vi "wsHandlerEngine.vi"(8 "error in (no error)":errorcluster, 11 "References":T1) -> (0 "error out":errorcluster)   [LabVIEW 2018, in "HASS-LV-WS_integration.lvlib"]
uses:
  HASS-LV-WS_integration.lvlib
  TypeDef/ReferencesTypeDef.ctl
  TypeDef/QueueTypeDef.ctl
  TypeDef/EventTypeDef.ctl
  TypeDef/registeredEventTypeDef.ctl
  <vilib>/MediaMongrels Ltd/WebSockets/WebSockets/WebSockets.lvlib
panel:
  out "error live":errorcluster
  out "eventMsgIDs":string[](array[string])
  out "Log":string
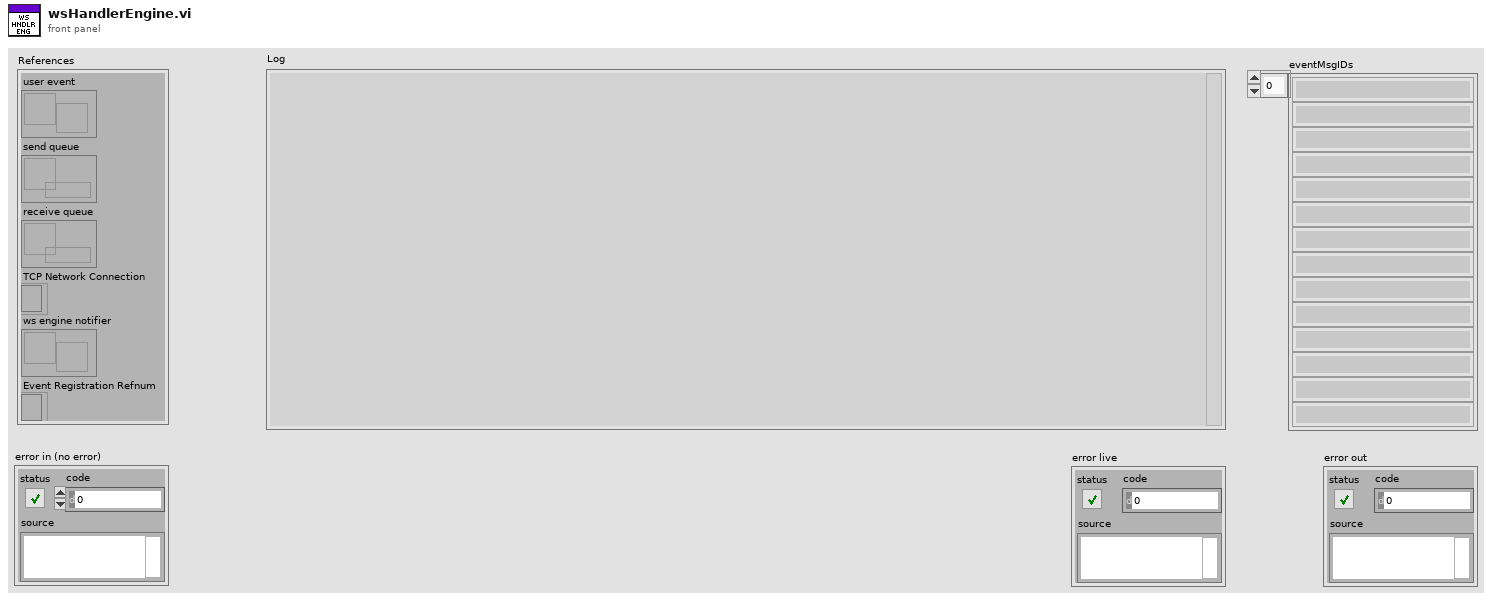
[diagram p1: front panel]
types:
  T1 = typedef "HASS-LV-WS_integration.lvlib/ReferencesTypeDef.ctl" = cluster{"user event":refnum<user-event>, "send queue":refnum<queue>, "receive queue":refnum<queue>, "TCP Network Connection":refnum<k5>, "ws engine notifier ":refnum<notifier>, "Event Registration Refnum":refnum<event-registration>}
  T2 = typedef "HASS-LV-WS_integration.lvlib/EventTypeDef.ctl" = cluster{"Data":variant, "Command":string}
  T3 = typedef "HASS-LV-WS_integration.lvlib/registeredEventTypeDef.ctl" = enum16{"Init", "Register", "Unregister", "Get MSG ID", "Get Event Name", "Get All Events"}
  T4 = typedef "HASS-LV-WS_integration.lvlib/QueueTypeDef.ctl" = cluster{"Data":variant, "Command":string}
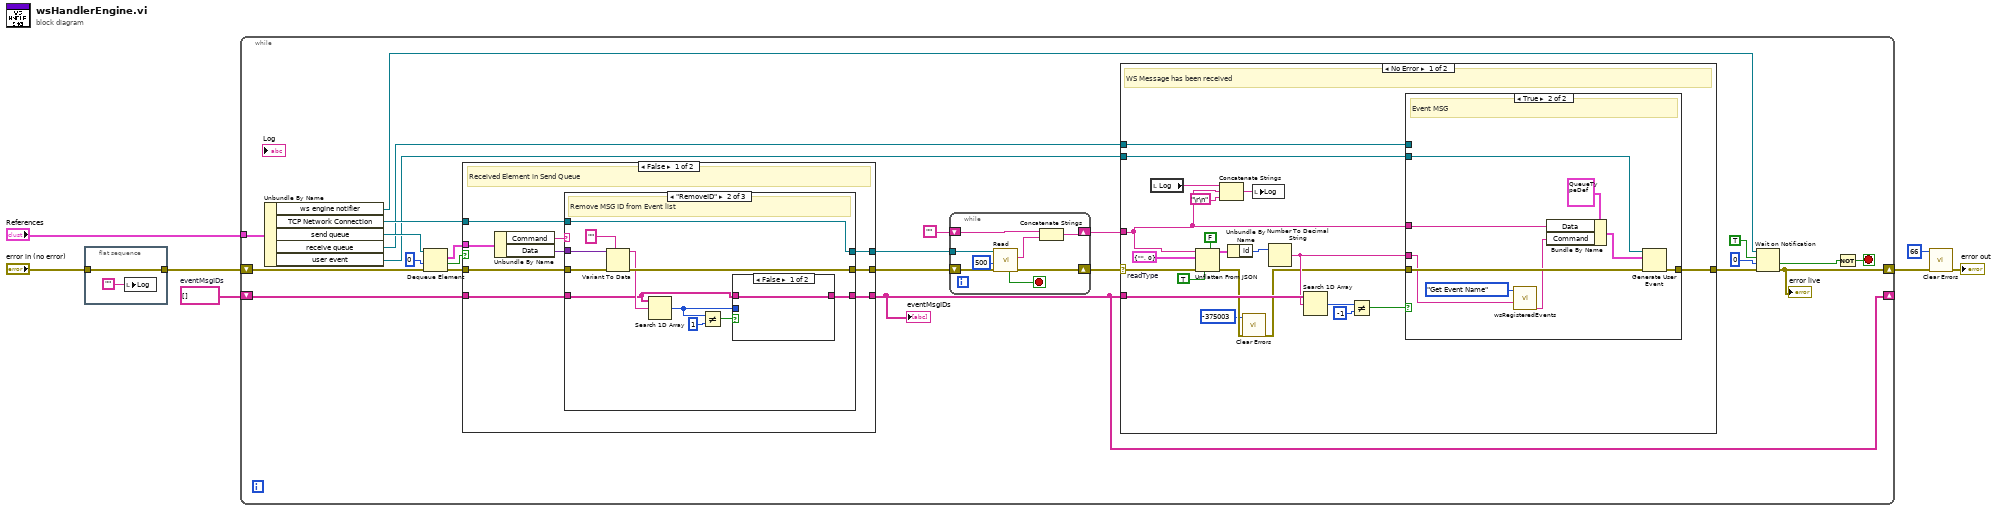
[diagram p0: block diagram]
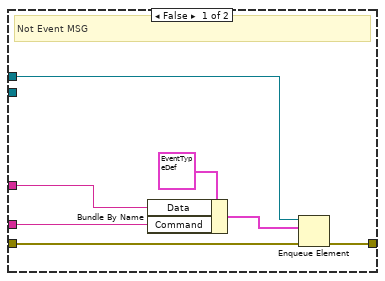
[diagram p2: hidden frame]
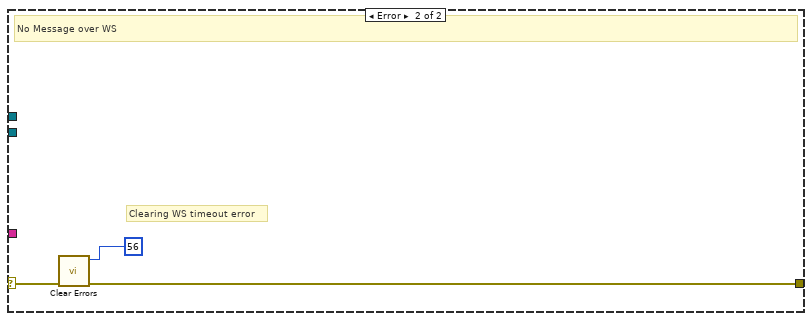
[diagram p3: hidden frame]
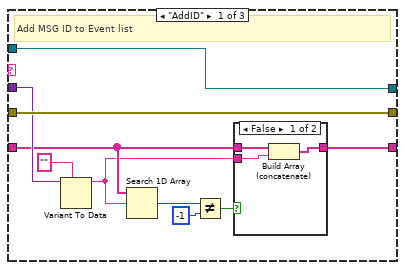
[diagram p4: hidden frame]
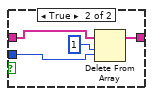
[diagram p6: hidden frame]
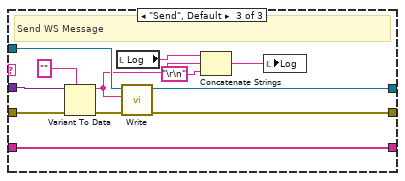
[diagram p7: hidden frame]
diagram:
  w7 = string[] []  # eventMsgIDs
  n1 = flat-sequence {
    tunnel: "error in (no error)" -> [w9]
    tunnel: [w9] -> w4
    frame #0 {
      n2 = local write "Log"("") -> ()
    }
  }
  n3 = while {
    tunnel: "References" -> [w33]
    shift-right: [w21] -> _
    shift-left: w7 -> [w23]
    shift-right: [w13] -> w3
    shift-left: w4 -> [w30]
    stop <- w15 stop-if-true
    n4 = Unbundle By Name(w33) -> ("ws engine notifier"=w18:refnum<notifier>, "TCP Network Connection"=w29:refnum<k5>, "send queue"=w32:refnum<queue>, "receive queue"=w19:refnum<queue>, "user event"=w20:refnum<user-event>)
    n5 = Dequeue Element(queue=w32, timeout in ms (-1)=0, error in (no error)=w30) -> (element=w26:T2, timed out?=w27:bool, error out=w28:errorcluster)  [unwired: 1 out]
    n6 = case shown="False" w27 {
      tunnel: w29 -> [w90 w134]
      tunnel: w28 -> [w89 w135]
      tunnel: w26 -> [w88 _]
      tunnel: [w86 w135] -> w25
      tunnel: [w85 w134] -> w24
      tunnel: w23 -> [w83 w133]
      tunnel: [w82 w133] -> w21
      frame False {
        # "Received Element in Send Queue"
        n7 = Unbundle By Name(w88) -> ("Command"=w84:string, "Data"=w87:variant)
        n8 = case shown="\"RemoveID\"" w84 {
          tunnel: w90 -> [w100 w115 w132]
          tunnel: w89 -> [w99 w113 w125]
          tunnel: w87 -> [w98 w114 w131]
          tunnel: [w99 w112 w129] -> w86
          tunnel: [w100 w115 w128] -> w85
          tunnel: w83 -> [w94 w109 w127]
          tunnel: [w91 w108 w127] -> w82
          frame "AddID" {
            # "Add MSG ID to Event list"
            n9 = Variant To Data(type="", Variant=w98) -> (data=w93:string)  [unwired: 1 in, 1 out]
            n10 = Search 1D Array(1D array=w94, element=w93) -> (index of element=w96:i32)  [unwired: 1 in]
            n11 = Not Equal?(x=w96, y=-1) -> (x != y?=w92:bool)
            n12 = case shown="False" w92 {
              tunnel: w94 -> [w103 w104]
              tunnel: w93 -> [w102 _]
              tunnel: [w101 w104] -> w91
              frame False {
                n13 = Build Array (concatenate)(w103, w102) -> (w101:string[])
              }
              frame True {
              }
            }
          }
          frame "RemoveID" {
            # "Remove MSG ID from Event list"
            n14 = Variant To Data(error in=w113, type="", Variant=w114) -> (data=w111:string, error out=w112:errorcluster)
            n15 = Search 1D Array(1D array=w109, element=w111) -> (index of element=w107:i32)  [unwired: 1 in]
            n16 = Not Equal?(x=w107, y=1) -> (x != y?=w105:bool)
            n17 = case shown="False" w105 {
              tunnel: w109 -> [w116 w120]
              tunnel: [w116 w119] -> w108
              tunnel: w107 -> [_ w117]
              frame False {
              }
              frame True {
                n18 = Delete From Array(array=w120, length=1, index=w117) -> (array with subset deleted=w119:string[])  [unwired: 1 out]
              }
            }
          }
          frame "Send", Default {
            # "Send WS Message"
            n19 = Variant To Data(error in=w125, type="", Variant=w131) -> (data=w121:string, error out=w126:errorcluster)
            n20 = local read "Log"() -> (w123:string)
            n21 = call <vilib>:"Write.vi"("error in (no error)"=w126, "Data"=w121, "WebSocket Connection in"=w132) -> ("error out"=w129:errorcluster, "WebSocket Connection out"=w128:refnum<k5>)  [unwired: 7 in]
            n22 = Concatenate Strings(w123, w121, "\r\n") -> (w124:string)
            n23 = local write "Log"(w124) -> ()
          }
        }
      }
      frame True {
        # "Send Queue Timed Out"
      }
    }
    "eventMsgIDs" <- w21
    n24 = while {
      tunnel: w24 -> [w40]
      shift-right: [w38] -> w22
      shift-left: w25 -> [w41]
      shift-right: [w36] -> w10
      shift-left: "" -> [w35]
      stop <- w37 stop-if-true
      n25 = call <vilib>:"Read.vi"("error in (no error)"=w41, "timeout ms (5000)"=500, "WebSocket Connection in"=w40) -> ("error out"=w38:errorcluster, "Data"=w34:string, "Finished?"=w37:bool)  [unwired: 4 in, 2 out]
      n26 = Concatenate Strings(w35, w34) -> (w36:string)
    }
    n27 = case shown="No Error" w22 {
      selector: w22 -> [w60 w81]
      tunnel: w10 -> [w49 _]
      tunnel: [w53 w80] -> w14
      tunnel: w21 -> [w59 _]
      tunnel: w20 -> [w55 _]
      tunnel: w19 -> [w54 _]
      frame No Error {
        w62 = cluster{"type":string, "id":i32} {"type"="", "id"=0}  # readType
        # "WS Message has been received"
        n28 = local read "Log"() -> (w51:string)
        n29 = Unflatten From JSON(enable LabVIEW extensions? (T)=FALSE, JSON string=w49, type and defaults=w62, default null elements? (F)=TRUE, error in (no error)=w60) -> (value=w61:cluster{"type":string, "id":i32}, error out=w44:errorcluster)  [unwired: 2 in]
        n30 = Concatenate Strings(w51, w49, "\r\n") -> (w50:string)
        n31 = Unbundle By Name(w61) -> ("id"=w48:i32)
        n32 = call <vilib>:"Clear Errors.vi"("error in (no error)"=w44, "specific error code to clear (0: all)"=-375003) -> ("error out"=w43:errorcluster)  [unwired: 4 in, 1 out]
        n33 = local write "Log"(w50) -> ()
        n34 = Number To Decimal String(number=w48) -> (decimal integer string=w47:string)  [unwired: 1 in]
        n35 = Search 1D Array(1D array=w59, element=w47) -> (index of element=w58:i32)  [unwired: 1 in]
        n36 = Not Equal?(x=w58, y=-1) -> (x != y?=w56:bool)
        n37 = case shown="True" w56 {
          tunnel: w55 -> [_ w78]
          tunnel: w43 -> [w68 w77]
          tunnel: w47 -> [w63 w72]
          tunnel: w54 -> [w69 _]
          tunnel: [w67 w74] -> w53
          tunnel: w49 -> [w64 w73]
          frame False {
            # "Not Event MSG"
            n38 = Bundle By Name(cluster=T2 {"Data"=variant, "Command"=""} ("element"), "Data"=w64, "Command"=w63) -> (w65:T2)
            n39 = Enqueue Element(queue=w69, element=w65, error in (no error)=w68) -> (error out=w67:errorcluster)  [unwired: 1 in, 2 out]
          }
          frame True {
            # "Event MSG"
            n40 = call "wsRegisteredEvents.vi"("msgID"=w72, "Action"=registeredEventTypeDef."Get Event Name") -> ("Event Name"=w71:string)  [unwired: 6 in, 3 out]
            n41 = Bundle By Name(cluster=T4 {"Data"=variant, "Command"=""} ("event data"), "Data"=w73, "Command"=w71) -> (w75:T4)
            n42 = Generate User Event(user event=w78, event data cluster=w75, error in=w77) -> (error out=w74:errorcluster)  [unwired: 1 in, 1 out]
          }
        }
      }
      frame Error {
        # "Clearing WS timeout error"
        # "No Message over WS"
        n43 = call <vilib>:"Clear Errors.vi"("error in (no error)"=w81, "specific error code to clear (0: all)"=56) -> ("error out"=w80:errorcluster)  [unwired: 4 in, 1 out]
      }
    }
    n44 = Wait on Notification(notifier=w18, ignore previous (F)=TRUE, timeout in ms (-1)=0, error in (no error)=w14) -> (timed out?=w16:bool, error out=w13:errorcluster)  [unwired: 2 out]
    "error live" <- w13
    n45 = Not(x=w16) -> (.not. x?=w15:bool)
  }
  n46 = call <vilib>:"Clear Errors.vi"("error in (no error)"=w3, "specific error code to clear (0: all)"=66) -> ("error out"=→"error out":errorcluster)  [unwired: 4 in, 1 out]
